vi "Switch Protection Signal.vi"(5 "Incoming Page GUID":string, 6 "Invalid Count Channel GUID":string, 7 "Protected Signal GUID":string, 8 "error in (no error)":errorcluster, 9 "Signal Page GUID":string, 10 "Protection Value GUID":string, 11 "Node Ptr":T1 format="%.0x") -> (0 "error out":errorcluster)   [LabVIEW 2023, in "Protection and Counter Support System Explorer.lvlib"]
uses:
  Protection and Counter Support System Explorer.lvlib
  <vilib>/NI VeriStand/Custom Device API/Custom Device Item Ref.ctl
  <vilib>/NI VeriStand/Custom Device API/Custom Device Channel.ctl
  <vilib>/NI VeriStand/Custom Device API/Custom Device Channel Type.ctl
  <vilib>/NI VeriStand/Custom Device API/Custom Device API.lvlib
  <vilib>/NI VeriStand/Custom Device Tools/Custom Device Utility Library/Custom Device Utility Library.lvlib
  f129ba6d-420f-49b5-9327-8e35f7b30b81.vi
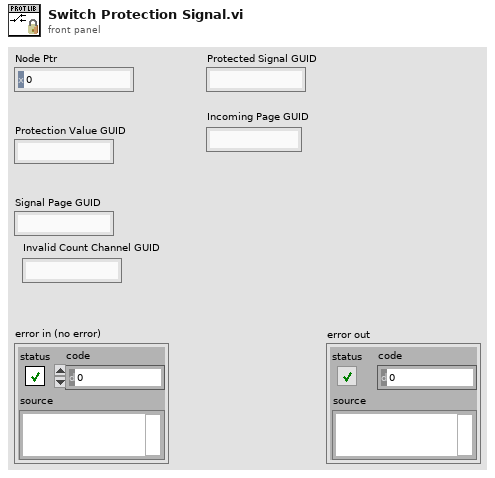
[diagram p1: front panel]
types:
  T1 = typedef "Custom Device API.lvlib/Custom Device Item Ref.ctl" = u64
  T2 = typedef "Custom Device API.lvlib/Custom Device Item Info.ctl" = cluster{"Name":string, "Is Channel":bool, "GUID":string, "Is Waveform":bool}
  T3 = typedef "Custom Device API.lvlib/Custom Device Channel.ctl" = cluster{"Type":T4, "Units":string, "Default Value":dbl, "Faultable":bool, "Scalable":bool}
  T4 = typedef "Custom Device API.lvlib/Custom Device Channel Type.ctl" = enum16{"Input", "Output"}
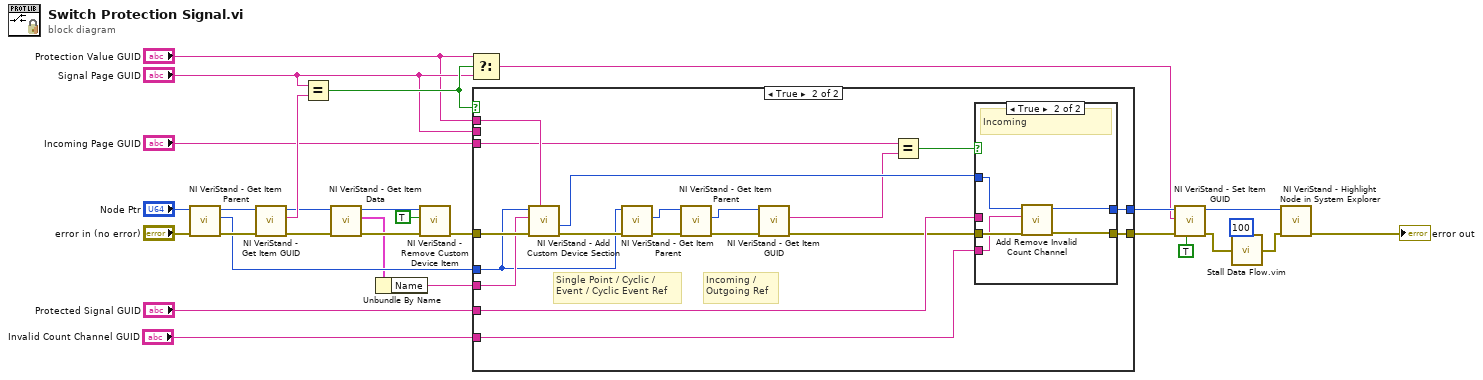
[diagram p0: block diagram]
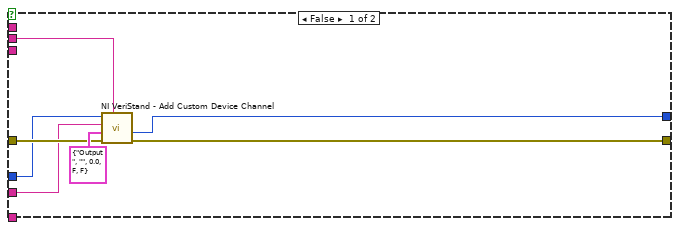
[diagram p2: hidden frame]
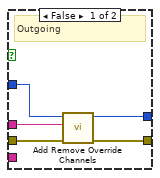
[diagram p3: hidden frame]
diagram:
  n1 = call <vilib>:"NI VeriStand - Get Item Parent.vi"("error in (no error)"="error in (no error)", "Item Ref in"="Node Ptr") -> ("error out"=w18:errorcluster, "Parent Ref"=w15:T1, "Item Ref out"=w20:T1)  [unwired: 6 in, 1 out]
  n2 = call <vilib>:"NI VeriStand - Get Item GUID.vi"("error in (no error)"=w18, "Item Ref in"=w20) -> ("error out"=w13:errorcluster, "GUID"=w24:string, "Item Ref out"=w17:T1)  [unwired: 7 in]
  n3 = Equal?(x="Signal Page GUID", y=w24) -> (x = y?=w22:bool)
  n4 = call <vilib>:"NI VeriStand - Get Item Data.vi"("error in (no error)"=w13, "Item Ref in"=w17) -> ("error out"=w12:errorcluster, "Item Info"=w11:T2, "Item Ref out"=w14:T1)  [unwired: 6 in, 1 out]
  n5 = Unbundle By Name(w11) -> ("Name"=w10:string)
  n6 = call <vilib>:"NI VeriStand - Remove Custom Device Item.vi"("error in (no error)"=w12, "Force Delete (F)"=TRUE, "Item Ref in"=w14) -> ("error out"=w16:errorcluster)  [unwired: 7 in, 1 out]
  n7 = Select(t="Protection Value GUID", s=w22, f="Signal Page GUID") -> (s? t:f=w26:string)
  n8 = case shown="True" w22 {
    tunnel: w16 -> [w35 w53]
    tunnel: [w31 w54] -> w28
    tunnel: w15 -> [w34 w42]
    tunnel: [w30 w48] -> w29
    tunnel: "Signal Page GUID" -> [w33 _]
    tunnel: w10 -> [w32 w49]
    tunnel: "Protected Signal GUID" -> [_ w51]
    tunnel: "Protection Value GUID" -> [_ w50]
    tunnel: "Invalid Count Channel GUID" -> [_ w38]
    tunnel: "Incoming Page GUID" -> [_ w37]
    frame False {
      n9 = call <vilib>:"NI VeriStand - Add Custom Device Channel.vi"("GUID (Default Channel)"=w33, "error in (no error)"=w35, "Channel"=T3 {"Type"=enum."Output", "Units"="", "Default Value"=0.0, "Faultable"=FALSE, "Scalable"=FALSE}, "Channel Name"=w32, "Parent Ref in"=w34) -> ("error out"=w31:errorcluster, "Channel Ref"=w30:T1)  [unwired: 3 in, 2 out]
    }
    frame True {
      # "Incoming / \nOutgoing Ref"
      # "Single Point / Cyclic / \nEvent / Cyclic Event Ref"
      n10 = call <vilib>:"NI VeriStand - Add Custom Device Section.vi"("GUID (Default Section)"=w50, "error in (no error)"=w53, "Section Name"=w49, "Parent Ref in"=w42) -> ("error out"=w44:errorcluster, "Section Ptr"=w52:T1)  [unwired: 4 in, 2 out]
      n11 = call <vilib>:"NI VeriStand - Get Item Parent.vi"("error in (no error)"=w44, "Item Ref in"=w42) -> ("error out"=w46:errorcluster, "Parent Ref"=w41:T1)  [unwired: 6 in, 2 out]
      n12 = call <vilib>:"NI VeriStand - Get Item Parent.vi"("error in (no error)"=w46, "Item Ref in"=w41) -> ("error out"=w45:errorcluster, "Parent Ref"=w40:T1)  [unwired: 6 in, 2 out]
      n13 = call <vilib>:"NI VeriStand - Get Item GUID.vi"("error in (no error)"=w45, "Item Ref in"=w40) -> ("error out"=w43:errorcluster, "GUID"=w39:string)  [unwired: 7 in, 1 out]
      n14 = Equal?(x=w37, y=w39) -> (x = y?=w47:bool)
      n15 = case shown="True" w47 {
        tunnel: [w59 w62] -> w54
        tunnel: w43 -> [w58 w61]
        tunnel: w52 -> [w57 w64]
        tunnel: w51 -> [w56 _]
        tunnel: [w55 w63] -> w48
        tunnel: w38 -> [_ w60]
        frame False {
          # "Outgoing"
          n16 = call "Add Remove Override Channels.vi"("error in (no error)"=w58, "Protected Signal GUID"=w56, "Channel Ref in"=w57) -> ("error out"=w59:errorcluster, "Channel Ref out"=w55:T1)  [unwired: 7 in]
        }
        frame True {
          # "Incoming"
          n17 = call "Add Remove Invalid Count Channel.vi"("error in (no error)"=w61, "Invalid Count Channel GUID"=w60, "Channel Ref in"=w64) -> ("error out"=w62:errorcluster, "Channel Ref out"=w63:T1)  [unwired: 7 in]
        }
      }
    }
  }
  n18 = call <vilib>:"NI VeriStand - Set Item GUID.vi"("Refresh System Explorer Tree? (F)"=TRUE, "error in (no error)"=w28, "GUID"=w26, "Item Ref in"=w29) -> ("error out"=w3:errorcluster, "Item Ref out"=w27:T1)  [unwired: 6 in]
  n19 = call "Stall Data Flow.vim"("value in"=w3, "milliseconds to wait"=u32 100) -> ("value out"=w2:errorcluster)  [unwired: 1 out]
  n20 = call <vilib>:"NI VeriStand - Highlight Node in System Explorer.vi"("error in (no error)"=w2, "Item Ref in"=w27) -> ("error out"=→"error out":errorcluster)  [unwired: 8 in, 1 out]
